vi "Get Y Min Voltage.vi"(8 "error in (no error)":errorcluster, 11 "hdl in":i32) -> (0 "error out":errorcluster, 2 "Get y min voltage(V)":dbl, 3 "hdl":i32)   [LabVIEW 2011, in "Thorlabs_MDT69xB.lvlib"]
doc: "Reads the minimum output voltage limit for Y axis."
uses:
  <instrlib>/Thorlabs_MDT69xB/Thorlabs_MDT69xB.lvlib
  <instrlib>/Thorlabs_MDT69xB/Data/MDT_COMMAND_LIB_win32.dll
  <instrlib>/Thorlabs_MDT69xB/Data/MDT_COMMAND_LIB_x64.dll
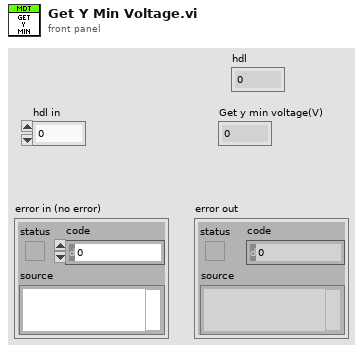
[diagram p1: front panel]
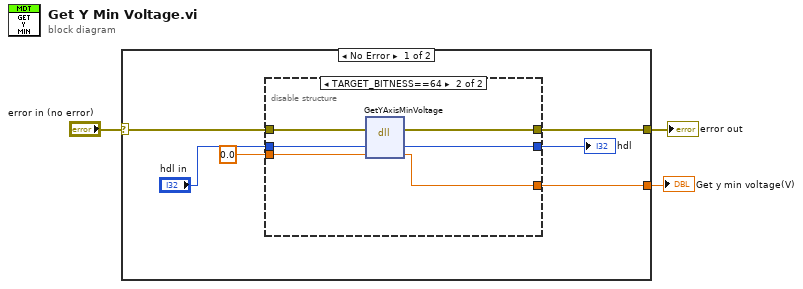
[diagram p0: block diagram]
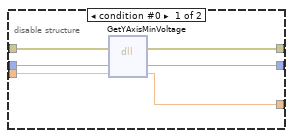
[diagram p2: hidden frame]
diagram:
  n1 = case shown="No Error" "error in (no error)" {
    selector: "error in (no error)" -> [w4 w22]
    tunnel: [w6 w22] -> w2
    tunnel: [w7 _] -> w1
    frame No Error {
      n2 = disable-structure shown="TARGET_BITNESS==64" {
        disable-tunnel: "hdl in" -> [w15 w21]
        disable-tunnel: 0.0 ("voltage") -> [w14 w20]
        disable-tunnel: [w13 w19] -> w7
        disable-tunnel: [w12 w18] -> w6
        disable-tunnel: [w11 w17] -> w5
        disable-tunnel: w4 -> [w10 w16]
        frame condition #0 {
          n3 = dll-call lib="E:/Program Files (x86)/National Instruments/LabVIEW 2011/instr.lib/Thorlabs_MDT69xB/Data/MDT_COMMAND_LIB_win32.dll" fn="GetYAxisMinVoltage"(error in=w10, "hdl"=w15, "voltage"=w14) -> (error out=w12:errorcluster, "hdl"=w11:i32, "voltage"=w13:dbl)  [unwired: 3 in, 1 out]
        }
        frame condition #1 (active) {
          n4 = dll-call lib="C:/Program Files/National Instruments/LabVIEW 2011/instr.lib/Thorlabs_MDT69xB/Data/MDT_COMMAND_LIB_x64.dll" fn="GetYAxisMinVoltage"(error in=w16, "hdl"=w21, "voltage"=w20) -> (error out=w18:errorcluster, "hdl"=w17:i32, "voltage"=w19:dbl)  [unwired: 3 in, 1 out]
        }
      }
      "hdl" <- w5
    }
    frame Error {
    }
  }
  "error out" <- w2
  "Get y min voltage(V)" <- w1
